vi "Set Message Protection.vi"(7 "Protection Type":T1, 8 "error in (no error)":errorcluster, 11 "Message in":T2 format="%.0x") -> (0 "error out":errorcluster, 3 "Message out":T2 format="%.0x")   [LabVIEW 2020, in "Instrument Addon Scripting API.lvlib"]
uses:
  Instrument Addon Scripting API.lvlib
  <vilib>/NI VeriStand/Custom Device API/Custom Device Item Ref.ctl
  TypeDefs/Protection Types.ctl
  Shared Directory/FG Control.ctl
  Shared Directory/Constants.vi
  <vilib>/NI VeriStand/Custom Device API/NI VeriStand - Get Item Property.vi
  <vilib>/NI VeriStand/Custom Device API/Get Item Property (U32).vi
  <vilib>/NI VeriStand/Custom Device API/Get Item Property (Double).vi
  <vilib>/NI VeriStand/Custom Device API/Get Item Property (Boolean).vi
  <vilib>/NI VeriStand/Custom Device API/Get Item Property (String).vi
  <vilib>/NI VeriStand/Custom Device API/NI VeriStand - Set Item Property.vi
  <vilib>/NI VeriStand/Custom Device API/Set Item Property (U32).vi
  <vilib>/NI VeriStand/Custom Device API/Set Item Property (Double).vi
  <vilib>/NI VeriStand/Custom Device API/Set Item Property (Boolean).vi
  <vilib>/NI VeriStand/Custom Device API/Set Item Property (String).vi
  Shared Directory/Instrument Addon Shared.lvlib
  <vilib>/NI VeriStand/Custom Device API/Custom Device API.lvlib
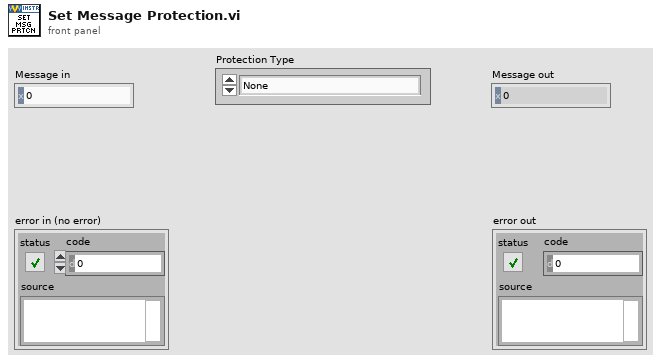
[diagram p1: front panel]
types:
  T1 = typedef "Instrument Addon Scripting API.lvlib/Protection Types.ctl" = enum16{"None", "CRC-32", "Checksum U16", "Checksum U32", "Checksum U8"}
  T2 = typedef "Custom Device API.lvlib/Custom Device Item Ref.ctl" = u64
  T3 = typedef "Instrument Addon Shared.lvlib/FG Control.ctl" = enum16{"Get", "Set"}
  T4 = typedef "Instrument Addon Shared.lvlib/Message Parameters.ctl" = cluster{"Generation Type":T5, "Period":dbl, "Include Protection":bool, "Type":string}
  T5 = typedef "Instrument Addon Shared.lvlib/Message Generation Type.ctl" = enum16{"Trigger Only", "Periodic & Trigger", "Value Change & Trigger"}
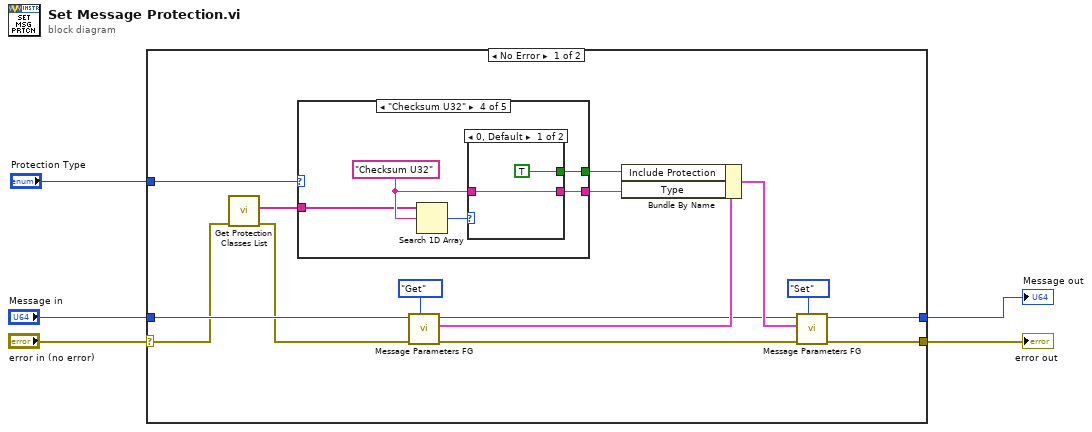
[diagram p0: block diagram]
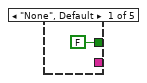
[diagram p2: hidden frame]
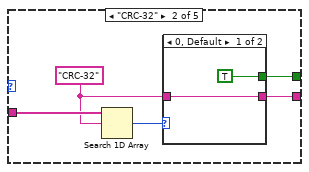
[diagram p3: hidden frame]
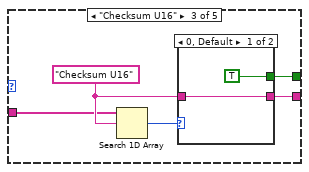
[diagram p5: hidden frame]
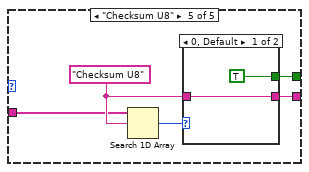
[diagram p8: hidden frame]
diagram:
  n1 = case shown="No Error" "error in (no error)" {
    selector: "error in (no error)" -> [w6 w51]
    tunnel: [w20 w50] -> w5
    tunnel: [w19 w51] -> w4
    tunnel: "Message in" -> [w18 w50]
    tunnel: "Protection Type" -> [w10 _]
    frame No Error {
      n2 = call "Get Protection Classes List.vi"("error in (no error)"=w6) -> ("error out"=w11:errorcluster, "Protection names"=w9:string[])  [unwired: 8 in, 1 out]
      n3 = case shown="\"Checksum U32\"" w10 {
        tunnel: w9 -> [_ w26 w29 w38 w45]
        tunnel: [_ w23 w31 w36 w43] -> w8
        tunnel: [FALSE ("Include Protection") w22 w30 w37 w44] -> w7
        frame "None", Default {
        }
        frame "CRC-32" {
          w24 = "CRC-32" ("element")
          n4 = Search 1D Array(1D array=w26, element=w24) -> (index of element=w25:i32)  [unwired: 1 in]
          n5 = case shown="0, Default" w25 {
            tunnel: w24 -> [w28 _]
            tunnel: [w28 _] -> w23
            tunnel: [TRUE ("Include Protection") _] -> w22
            frame 0, Default {
            }
            frame -1 {
            }
          }
        }
        frame "Checksum U16" {
          w32 = "Checksum U16" ("element")
          n6 = Search 1D Array(1D array=w29, element=w32) -> (index of element=w33:i32)  [unwired: 1 in]
          n7 = case shown="0, Default" w33 {
            tunnel: w32 -> [w35 _]
            tunnel: [w35 _] -> w31
            tunnel: [TRUE ("Include Protection") _] -> w30
            frame 0, Default {
            }
            frame -1 {
            }
          }
        }
        frame "Checksum U32" {
          w39 = "Checksum U32" ("element")
          n8 = Search 1D Array(1D array=w38, element=w39) -> (index of element=w40:i32)  [unwired: 1 in]
          n9 = case shown="0, Default" w40 {
            tunnel: w39 -> [w42 _]
            tunnel: [w42 _] -> w36
            tunnel: [TRUE ("Include Protection") _] -> w37
            frame 0, Default {
            }
            frame -1 {
            }
          }
        }
        frame "Checksum U8" {
          w46 = "Checksum U8" ("element")
          n10 = Search 1D Array(1D array=w45, element=w46) -> (index of element=w47:i32)  [unwired: 1 in]
          n11 = case shown="0, Default" w47 {
            tunnel: w46 -> [w49 _]
            tunnel: [w49 _] -> w43
            tunnel: [TRUE ("Include Protection") _] -> w44
            frame 0, Default {
            }
            frame -1 {
            }
          }
        }
      }
      n12 = call "Message Parameters FG.vi"("Action"=FG_Control."Get", "error in (no error)"=w11, "Item Ref in"=w18) -> ("error out"=w12:errorcluster, "Message Settings out"=w15:T4, "Item Ref out"=w13:T2)  [unwired: 6 in]
      n13 = Bundle By Name(cluster=w15, "Include Protection"=w7, "Type"=w8) -> (w16:T4)
      n14 = call "Message Parameters FG.vi"("Action"=FG_Control."Set", "error in (no error)"=w12, "Message Settings"=w16, "Item Ref in"=w13) -> ("error out"=w19:errorcluster, "Item Ref out"=w20:T2)  [unwired: 5 in, 1 out]
    }
    frame Error {
    }
  }
  "Message out" <- w5
  "error out" <- w4
